vi "2 mission_interpreter.vi"() -> ()   [LabVIEW 2011]
uses:
  2 Typedefs/UTM Location.ctl
  2 Classes/Mission/Mission.lvclass
  2 Classes/Waypoint/Waypoint.lvclass
  2 Globals/2 Global.vi
  2 Classes/MissionQueue/MissionQueue.lvclass
panel:
  out "Coords 2":T1 {"North" format="%#_10f"; "East" format="%#_8f"}
  in  "Buoy SE":T1 {"North" format="%#_10f"; "East" format="%#_8f"}
  in  "Buoy SW":T1 {"North" format="%#_10f"; "East" format="%#_8f"}
  in  "Buoy NW":T1 {"North" format="%#_10f"; "East" format="%#_8f"}
  in  "Buoy NE":T1 {"North" format="%#_10f"; "East" format="%#_8f"}
  out "Midpoint":T1 {"North" format="%#_10f"; "East" format="%#_8f"}
  out "Coords":T1 {"North" format="%#_10f"; "East" format="%#_8f"}
  out "Mission Type":T2(ring)
  # "TEST"
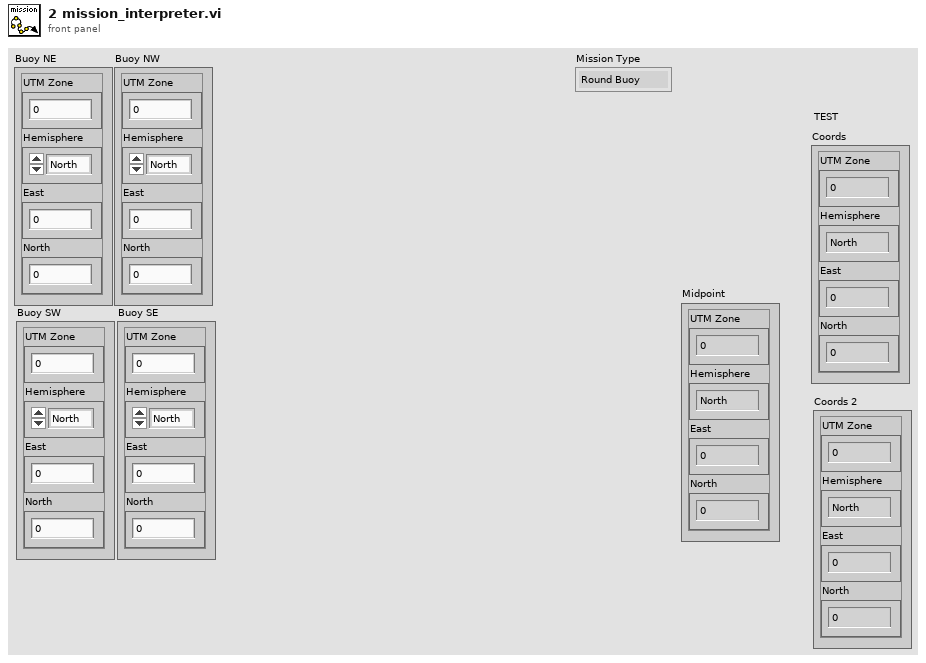
[diagram p1: front panel]
types:
  T1 = typedef "UTM Location.ctl" = cluster{"UTM Zone":dbl, "Hemisphere":enum16{"North", "South"}, "East":dbl, "North":dbl}
  T2 = enum16{"Round Buoy", "Drive", "Pass Buoys", "Station Keeping"}
  T3 = typedef "UTM Circle.ctl" = cluster{"UTM Zone":dbl, "Hemisphere":enum16{"North", "South"}, "East":dbl, "North":dbl, "Radius":dbl}
  T4 = typedef "Waypoints List.ctl" = refnum<class "Waypoint.lvclass">[]
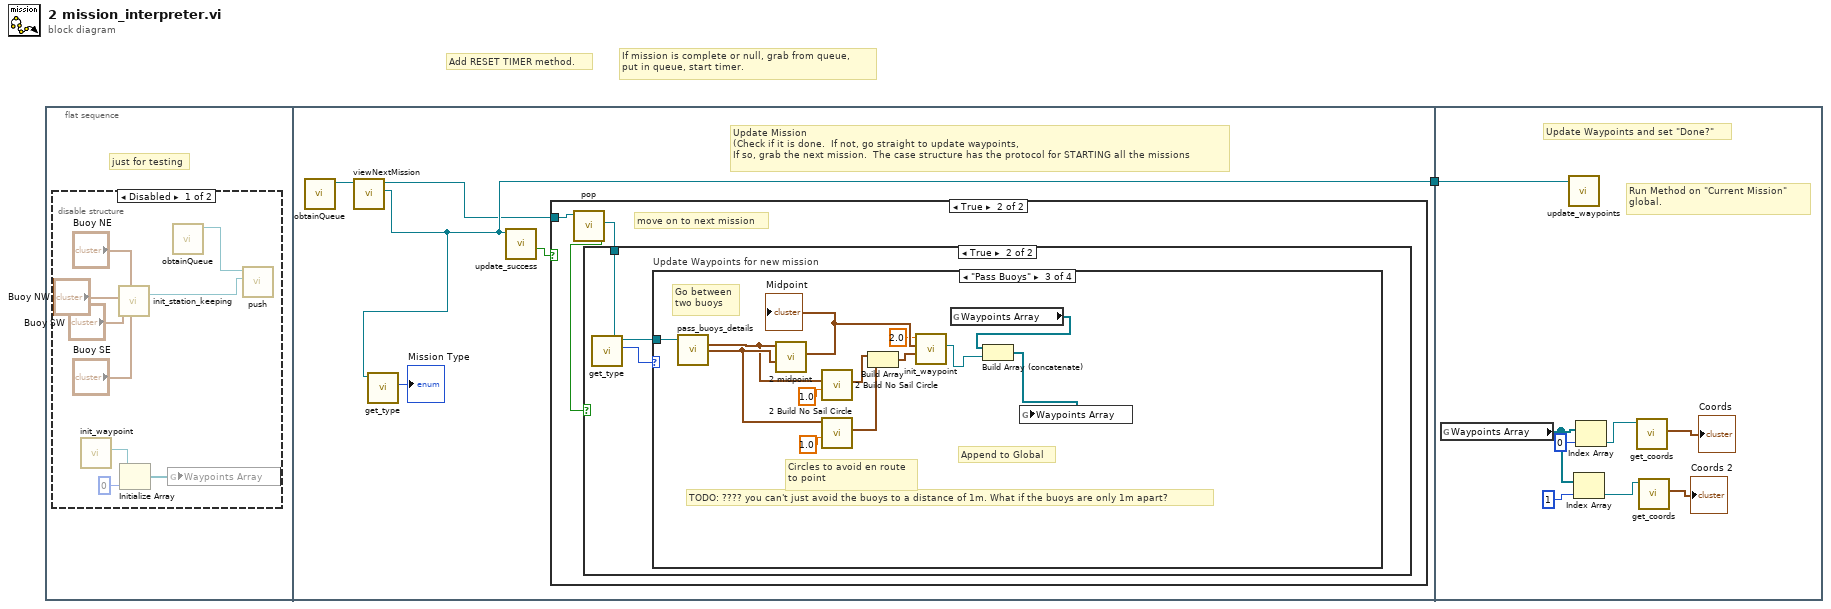
[diagram p0: block diagram]
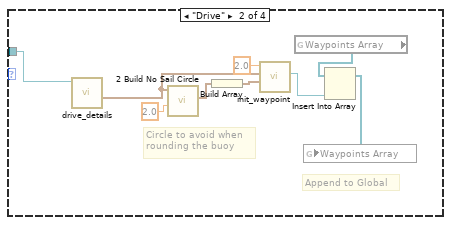
[diagram p6: hidden frame]
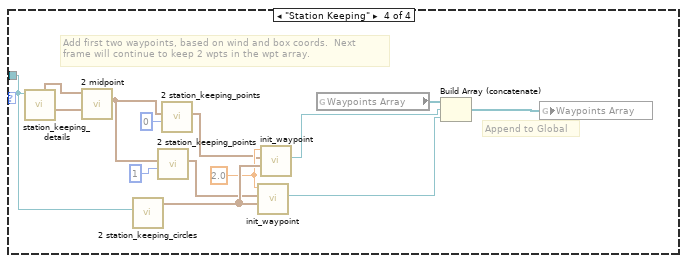
[diagram p7: hidden frame]
diagram:
  # "If mission is complete or null, grab from queue, \nput in queue, start timer."
  # "Add RESET TIMER method."
  n1 = flat-sequence {
    tunnel: [w13] -> w1
    tunnel: w1 -> [w65]
    frame #0 {
      # "just for testing"
      n2 = disable-structure shown="Disabled" {
        frame Disabled {
          n3 = call "init_waypoint.vi"() -> ("Waypoint Out"=w3:refnum<class "Waypoint.lvclass">)  [unwired: 11 in]
          n4 = call "init_station_keeping.vi"("Buoy SE"="Buoy SE", "Buoy NE"="Buoy NE", "Buoy SW"="Buoy SW", "Buoy NW"="Buoy NW") -> ("Mission out"=w9:refnum<class "Mission.lvclass">)  [unwired: 7 in]
          n5 = Initialize Array(w3, 0 ("dimension size")) -> (w4:refnum<class "Waypoint.lvclass">[])
          n6 = global write "2 Global.vi" "Waypoints Array"(w4) -> ()
          n7 = call "obtainQueue.vi"() -> ("MissionQueue.lvclass"=w10:refnum<class "MissionQueue.lvclass">)  [unwired: 10 in, 1 out]
          n8 = call "push.vi"("Mission.lvclass"=w9, "MissionQueue in"=w10) -> ()  [unwired: 8 in, 2 out]
        }
        frame Enabled {
        }
      }
    }
    frame #1 {
      # "Update Mission\n(Check if it is done.  If not, go straight to update waypoints,\nIf so, grab the next mission.  The case structure has the protocol for STARTING all the missions"
      n9 = call "obtainQueue.vi"() -> ("MissionQueue.lvclass"=w12:refnum<class "MissionQueue.lvclass">)  [unwired: 10 in, 1 out]
      n10 = call "viewNextMission.vi"("MissionQueue in"=w12) -> ("Mission.lvclass"=w13:refnum<class "Mission.lvclass">, "MissionQueue out"=w11:refnum<class "MissionQueue.lvclass">)  [unwired: 7 in, 2 out]
      n11 = call-dynamic "get_type.vi"("Mission in"=w13) -> ("Mission Type"=→"Mission Type":T2)  [unwired: 8 in, 2 out]
      n12 = call-dynamic "update_success.vi"("Mission in"=w13) -> ("Done?"=w15:bool)  [unwired: 9 in, 1 out]
      n13 = case shown="True" w15 {
        tunnel: w11 -> [_ w17]
        frame False {
        }
        frame True {
          # "move on to next mission"
          n14 = call "pop.vi"("MissionQueue in"=w17) -> ("Valid?"=w16:bool, "Mission.lvclass"=w18:refnum<class "Mission.lvclass">)  [unwired: 7 in, 2 out]
          n15 = case shown="True" w16 {
            tunnel: w18 -> [_ w20]
            frame False {
              # "no more valid missions."
            }
            frame True {
              n16 = call-dynamic "get_type.vi"("Mission in"=w20) -> ("Mission Type"=w21:T2, "Mission out"=w19:refnum<class "Mission.lvclass">)  [unwired: 8 in, 1 out]
              n17 = case "Update Waypoints for new mission" shown="\"Pass Buoys\"" w21 {
                tunnel: w19 -> [_ w24 w38 w52]
                frame "Round Buoy", Default {
                }
                frame "Drive" {
                  # "Append to Global"
                  # "Circle to avoid when\nrounding the buoy"
                  n18 = call-dynamic "drive_details.vi"("Mission in"=w24) -> ("Drive Location"=w23:T1)  [unwired: 9 in, 1 out]
                  n19 = call "2 Build No Sail Circle.vi"("Radius"=2.0, "UTM Location"=w23) -> ("UTM Circle"=w29:T3)  [unwired: 9 in]
                  n20 = Build Array(w29) -> (w30:T3[])
                  n21 = call "init_waypoint.vi"("No Sail Circles"=w30, "Coords"=w23, "Tolerance (m)"=2.0 ("Tolerance (meters?)")) -> ("Waypoint Out"=w22:refnum<class "Waypoint.lvclass">)  [unwired: 8 in]
                  n22 = global read "2 Global.vi" "Waypoints Array"() -> (w25:T4)
                  n23 = Insert Into Array(array=w25, new element=w22) -> (w26:T4)  [unwired: 1 in]
                  n24 = global write "2 Global.vi" "Waypoints Array"(w26) -> ()
                }
                frame "Pass Buoys" {
                  # "TODO: ???? you can't just avoid the buoys to a distance of 1m. What if the buoys are only 1m apart?"
                  # "Go between\ntwo buoys"
                  # "Append to Global"
                  # "Circles to avoid en route\nto point"
                  n25 = call-dynamic "pass_buoys_details.vi"("Mission in"=w38) -> ("Buoy Pass 1"=w34:T1, "Buoy Pass 2"=w35:T1)  [unwired: 11 in, 2 out]
                  n26 = call "2 midpoint.vi"("UTM 2"=w35, "UTM 1"=w34) -> ("Midpoint"=w41:T1)  [unwired: 9 in]
                  "Midpoint" <- w41
                  n27 = call "2 Build No Sail Circle.vi"("Radius"=1.0, "UTM Location"=w34) -> ("UTM Circle"=w42:T3)  [unwired: 9 in]
                  n28 = call "2 Build No Sail Circle.vi"("Radius"=1.0, "UTM Location"=w35) -> ("UTM Circle"=w37:T3)  [unwired: 9 in]
                  n29 = Build Array(w42, w37) -> (w43:T3[])
                  n30 = call "init_waypoint.vi"("No Sail Circles"=w43, "Coords"=w41, "Tolerance (m)"=2.0 ("Tolerance (meters?)")) -> ("Waypoint Out"=w31:refnum<class "Waypoint.lvclass">)  [unwired: 8 in]
                  n31 = global read "2 Global.vi" "Waypoints Array"() -> (w33:T4)
                  n32 = Build Array (concatenate)(w33, w31) -> (w32:T4)
                  n33 = global write "2 Global.vi" "Waypoints Array"(w32) -> ()
                }
                frame "Station Keeping" {
                  w50 = 2.0 ("Tolerance (meters?)")
                  # "Append to Global"
                  # "Add first two waypoints, based on wind and box coords.  Next\nframe will continue to keep 2 wpts in the wpt array."
                  n34 = call-dynamic "station_keeping_details.vi"("Mission in"=w52) -> ("Buoy SE"=w56:T1, "Buoy NW"=w57:T1)  [unwired: 4 in, 5 out]
                  n35 = call "2 midpoint.vi"("UTM 2"=w56, "UTM 1"=w57) -> ("Midpoint"=w47:T1)  [unwired: 9 in]
                  n36 = call "2 station_keeping_circles.vi"("Mission in"=w52) -> ("No Sail Circles"=w51:T3[])  [unwired: 10 in]
                  n37 = call "2 station_keeping_points.vi"("Which Point?"=1, "Midpoint"=w47) -> ("Waypoint"=w49:T1)  [unwired: 9 in]
                  n38 = call "2 station_keeping_points.vi"("Which Point?"=0, "Midpoint"=w47) -> ("Waypoint"=w48:T1)  [unwired: 9 in]
                  n39 = call "init_waypoint.vi"("No Sail Circles"=w51, "Coords"=w49, "Tolerance (m)"=w50) -> ("Waypoint Out"=w53:refnum<class "Waypoint.lvclass">)  [unwired: 8 in]
                  n40 = call "init_waypoint.vi"("No Sail Circles"=w51, "Coords"=w48, "Tolerance (m)"=w50) -> ("Waypoint Out"=w54:refnum<class "Waypoint.lvclass">)  [unwired: 8 in]
                  n41 = global read "2 Global.vi" "Waypoints Array"() -> (w55:T4)
                  n42 = Build Array (concatenate)(w55, w54, w53) -> (w44:T4)
                  n43 = global write "2 Global.vi" "Waypoints Array"(w44) -> ()
                }
              }
            }
          }
        }
      }
    }
    frame #2 {
      # "Run Method on \"Current Mission\"\nglobal."
      # "Update Waypoints and set \"Done?\""
      n44 = global read "2 Global.vi" "Waypoints Array"() -> (w60:T4)
      n45 = call-dynamic "update_waypoints.vi"("Mission in"=w65) -> ()  [unwired: 10 in, 1 out]
      n46 = Index Array(array=w60, index=1) -> (element=w61:refnum<class "Waypoint.lvclass">)
      n47 = Index Array(array=w60, index=0) -> (element=w64:refnum<class "Waypoint.lvclass">)
      n48 = call-dynamic "get_coords.vi"("Waypoint in"=w64) -> ("Coords"=→"Coords":T1)  [unwired: 7 in, 3 out]
      n49 = call-dynamic "get_coords.vi"("Waypoint in"=w61) -> ("Coords"=→"Coords 2":T1)  [unwired: 7 in, 3 out]
    }
  }
